vi "AFM_Litho_Plugin.IV.IVRun--Local.vi"(8 "error in (no error)":errorcluster, 10 "IV Run--Local":T1={"Pattern"=enum."Ramp /", "Cycles"=0.0, "Rate"=1.0, "End"=1.0, "Start"=0.0}, 11 "MeasurementSMO":refnum<class "AFM_Litho_Plugin.IV.lvclass">) -> (0 "error out":errorcluster, 3 "MeasurementSMO out":refnum<class "AFM_Litho_Plugin.IV.lvclass">)   [LabVIEW 2019, in "AFM_Litho_Plugin.IV.lvclass"]
doc: "---------------------------------------------------------------\nJKI State Machine Objects™\nhttp://jki.net/state-machine-objects/\nCopyright (C) 2005-2015, JKI <info@jki.net>\nALL RIGHTS RESERVEDJKI State Machine Objects (SMO) 1.0.0.4\nJKI - JKI\nCopyright (c) 2015, JKI"
uses:
  AFM_Litho_Plugin.IV.lvclass
  Typedefs/PrivateEvents--AFM_Litho_Plugin.IV.IV Run--Local.ctl
panel:
  # "For instructions on how to use the JKI State Machine Objects, examples and video tutorials, visit:\nhttp://jki.net/state-machine-objects/\n\nJKI State Machine Objects™\nhttp://jki.net/state-machine-objects/\nCopyright (C) 2005-2015, JKI <info@jki.net>\nALL RIGHTS RESERVED"
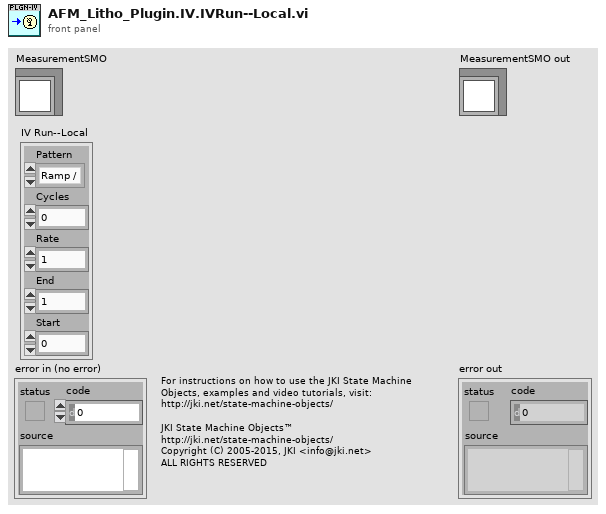
[diagram p1: front panel]
types:
  T1 = typedef "AFM_Litho_Plugin.IV.lvclass/PrivateEvents--AFM_Litho_Plugin.IV.IV Run--Local.ctl" = cluster{"Pattern":enum16{"Ramp /", "Ramp /\\", "Smooth Ramp _/", "Smooth Ramp _/\\_", "Frequency"}, "Cycles":dbl, "Rate":dbl, "End":dbl, "Start":dbl}
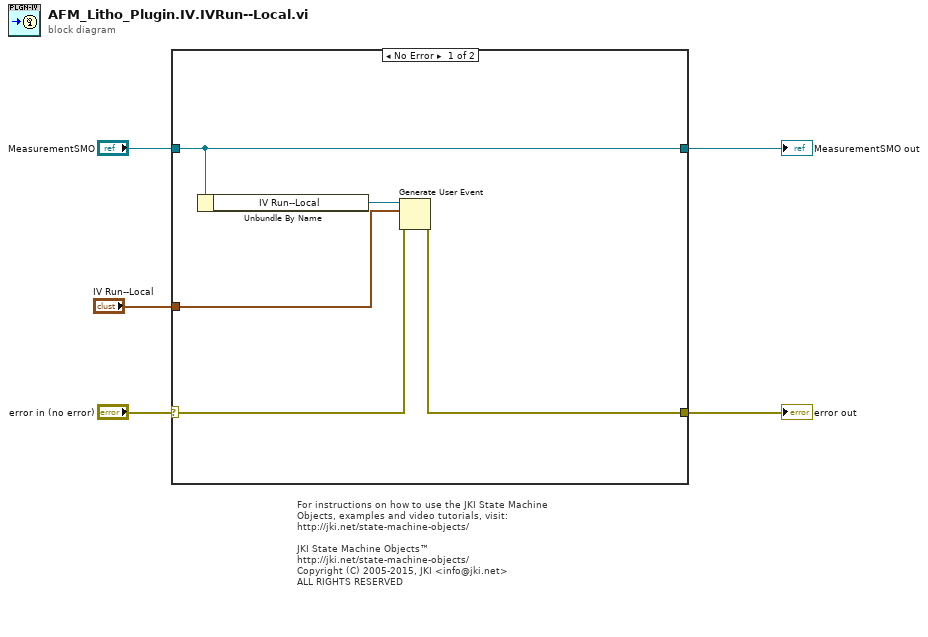
[diagram p0: block diagram]
diagram:
  # "For instructions on how to use the JKI State Machine Objects, examples and video tutorials, visit:\nhttp://jki.net/state-machine-objects/\n\nJKI State Machine Objects™\nhttp://jki.net/state-machine-objects/\nCopyright (C) 2005-2015, JKI <info@jki.net>\nALL RIGHTS RESERVED"
  n1 = case shown="No Error" "error in (no error)" {
    selector: "error in (no error)" -> [w10 w12]
    tunnel: [w7 w12] -> w4
    tunnel: [w6 w11] -> w5
    tunnel: "MeasurementSMO" -> [w6 w11]
    tunnel: "IV Run--Local" -> [w9 _]
    frame No Error {
      n2 = Unbundle By Name(w6) -> ("IV Run--Local"=w8:refnum<user-event>)
      n3 = Generate User Event(user event=w8, event data cluster=w9, error in=w10) -> (error out=w7:errorcluster)  [unwired: 1 in, 1 out]
    }
    frame Error {
    }
  }
  "error out" <- w4
  "MeasurementSMO out" <- w5
